vi "BIO_new_ssl.vi"(8 "error in (no error)":errorcluster, 10 "Client? (F=Server)":bool, 11 "SSL-Context in":refnum<class "SSL-Context.lvclass">) -> (0 "error out":errorcluster, 2 "SSL BIO out":refnum<class "BIO.lvclass">, 3 "SSL-Context out":refnum<class "SSL-Context.lvclass">)   [LabVIEW 2013, in "SSL_Lib.lvlib" / "SSL-Context.lvclass"]
uses:
  SSL-Context.lvclass
  BIO/BIO.lvclass
  SSL-Lib/SSL-Lib.lvclass/SSL-Lib.ctl
  SSL-Context.lvclass/SSL-Context.ctl
  BIO/BIO.lvclass/BIO.ctl
  SSL-Lib/Read SSL Library Path.vi
  Read Handle.vi
  BIO/Write Handle.vi
  SSL-Lib/SSL-Lib.lvclass
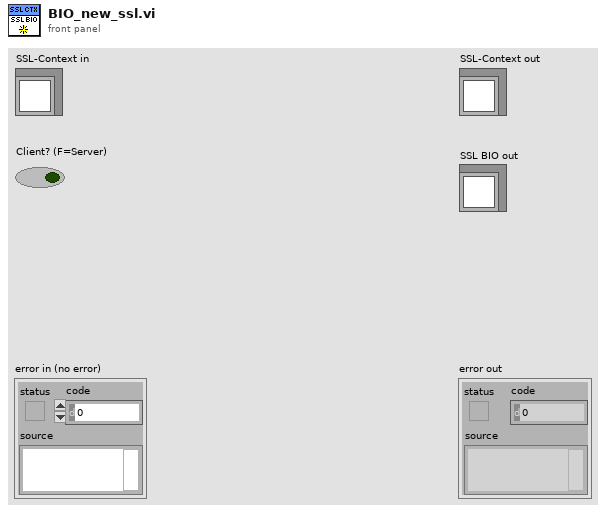
[diagram p1: front panel]
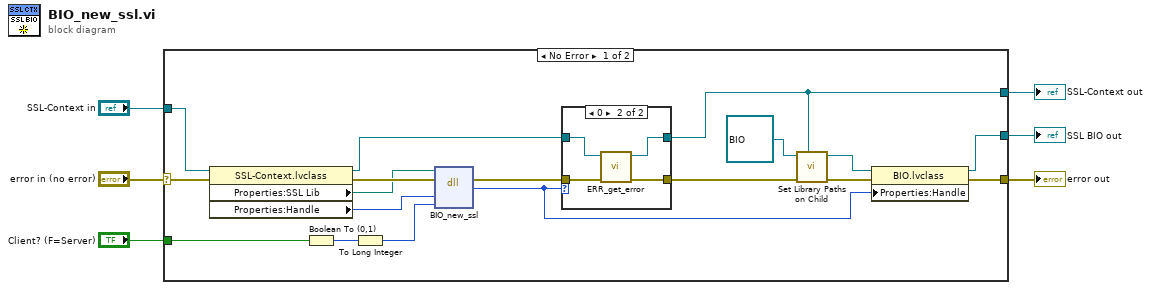
[diagram p0: block diagram]
diagram:
  n1 = case shown="No Error" "error in (no error)" {
    selector: "error in (no error)" -> [w24 w32]
    tunnel: [w16 w32] -> w5
    tunnel: [w12 w31] -> w3
    tunnel: "SSL-Context in" -> [w22 w31]
    tunnel: [w15 _] -> w2
    tunnel: "Client? (F=Server)" -> [w9 _]
    frame No Error {
      n2 = property class="SSL-Context.lvclass"(reference=w22, error in=w24) -> (reference out=w13:refnum<class "SSL-Context.lvclass">, error out=w23:errorcluster, "Properties:SSL Lib"=w21:path, "Properties:Handle"=w20:u64)
      n3 = Boolean To (0,1)(Boolean=w9) -> (0, 1=w8:i16)
      n4 = To Long Integer(number=w8) -> (32bit integer=w7:i32)
      n5 = dll-call lib="C:/Program Files (x86)/National Instruments/Shared/nissl/NIssleay32.dll" fn="BIO_new_ssl"(path in=w21, error in=w23, "SSL_CTX"=w20, "client"=w7) -> (error out=w14:errorcluster, "return type"=w10:u64)  [unwired: 3 in, 1 out]
      n6 = case shown="0" w10 {
        tunnel: w14 -> [w26 w30]
        tunnel: w13 -> [w25 w29]
        tunnel: [w25 w28] -> w12
        tunnel: [w26 w27] -> w11
        frame Default {
        }
        frame 0 {
          n7 = call "ERR_get_error.vi"("error in (no error)"=w30, "SSL-Lib in"=w29) -> ("error out"=w27:errorcluster, "SSL-Lib out"=w28:refnum<class "SSL-Context.lvclass">)  [unwired: 8 in]
        }
      }
      n8 = call-dynamic "Set Library Paths on Child.vi"(7:"SSL-Lib in"=w12, "error in (no error)"=w11, 11:"SSL-Lib in"=refnum<class "BIO.lvclass"> refnum ("SSL_Lib.lvlib:BIO.lvclass")) -> ("error out"=w18:errorcluster, "SSL-Lib out"=w17:refnum<class "BIO.lvclass">)  [unwired: 7 in]
      n9 = property class="BIO.lvclass"(reference=w17, error in=w18, "Properties:Handle"=w10) -> (reference out=w15:refnum<class "BIO.lvclass">, error out=w16:errorcluster)
    }
    frame Error {
    }
  }
  "error out" <- w5
  "SSL-Context out" <- w3
  "SSL BIO out" <- w2
